vi "Initialize Time Tab.vi"(8 "error in (no error)":errorcluster, 11 "Numeric Data Type in":refnum<class "Numeric Data Type.lvclass">) -> (0 "error out":errorcluster, 3 "Numeric Data Type (dub)":refnum<class "Numeric Data Type.lvclass">)   [LabVIEW 2018, in "Numeric Data Type.lvclass"]
uses:
  Numeric Data Type.lvclass
  Numeric Data Type.lvclass/Numeric Data Type.ctl
  Reference Time Format.vi
  Reference Include Seconds.vi
  Reference HMS Digits.vi
  Reference Clock Type.vi
  Reference Date Format.vi
  Reference Date Order.vi
  Reference Year Format.vi
  Reference Display Type.vi
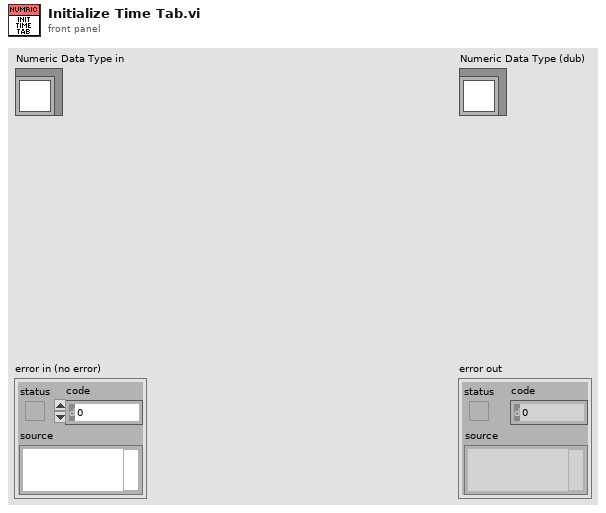
[diagram p1: front panel]
types:
  T1 = typedef "Numeric Data Type.lvclass/Time Info.ctl" = cluster{"Time Format":T2, "Numeric Format":T3, "Clock Type":T4, "Include Seconds?":bool, "Seconds Precision":i16, "Date Order":T5, "Date Format":T6, "Year Format":T7, "UTC":i16}
  T2 = typedef "Numeric Data Type.lvclass/Time Format.ctl" = enum16{"Custom time format", "System time format", "Time unused"}
  T3 = typedef "Numeric Data Type.lvclass/Numeric Format Enum.ctl" = enum16{"Floating Point Notation", "Scientific Notation", "Engineering Notation", "SI Notation", "<not used>", "Decimal", "Hexadecimal", "Octal", "Binary", "<not used 2>", "Absolute Time", "Relative Time"}
  T4 = typedef "Numeric Data Type.lvclass/Clock Type.ctl" = enum32{"12-Hour (AM/PM)", "24-Hour"}
  T5 = typedef "Numeric Data Type.lvclass/Date Order.ctl" = enum32{"M/D/Y", "D/M/Y", "Y/M/D"}
  T6 = typedef "Numeric Data Type.lvclass/Date Format.ctl" = enum16{"Custom date format", "System date format", "Date unused"}
  T7 = typedef "Numeric Data Type.lvclass/Year Format.ctl" = enum32{"No Year", "2-digit Year", "4-digit Year"}
  T8 = enum8{"Enabled", "Disabled", "Disabled and Grayed Out"}
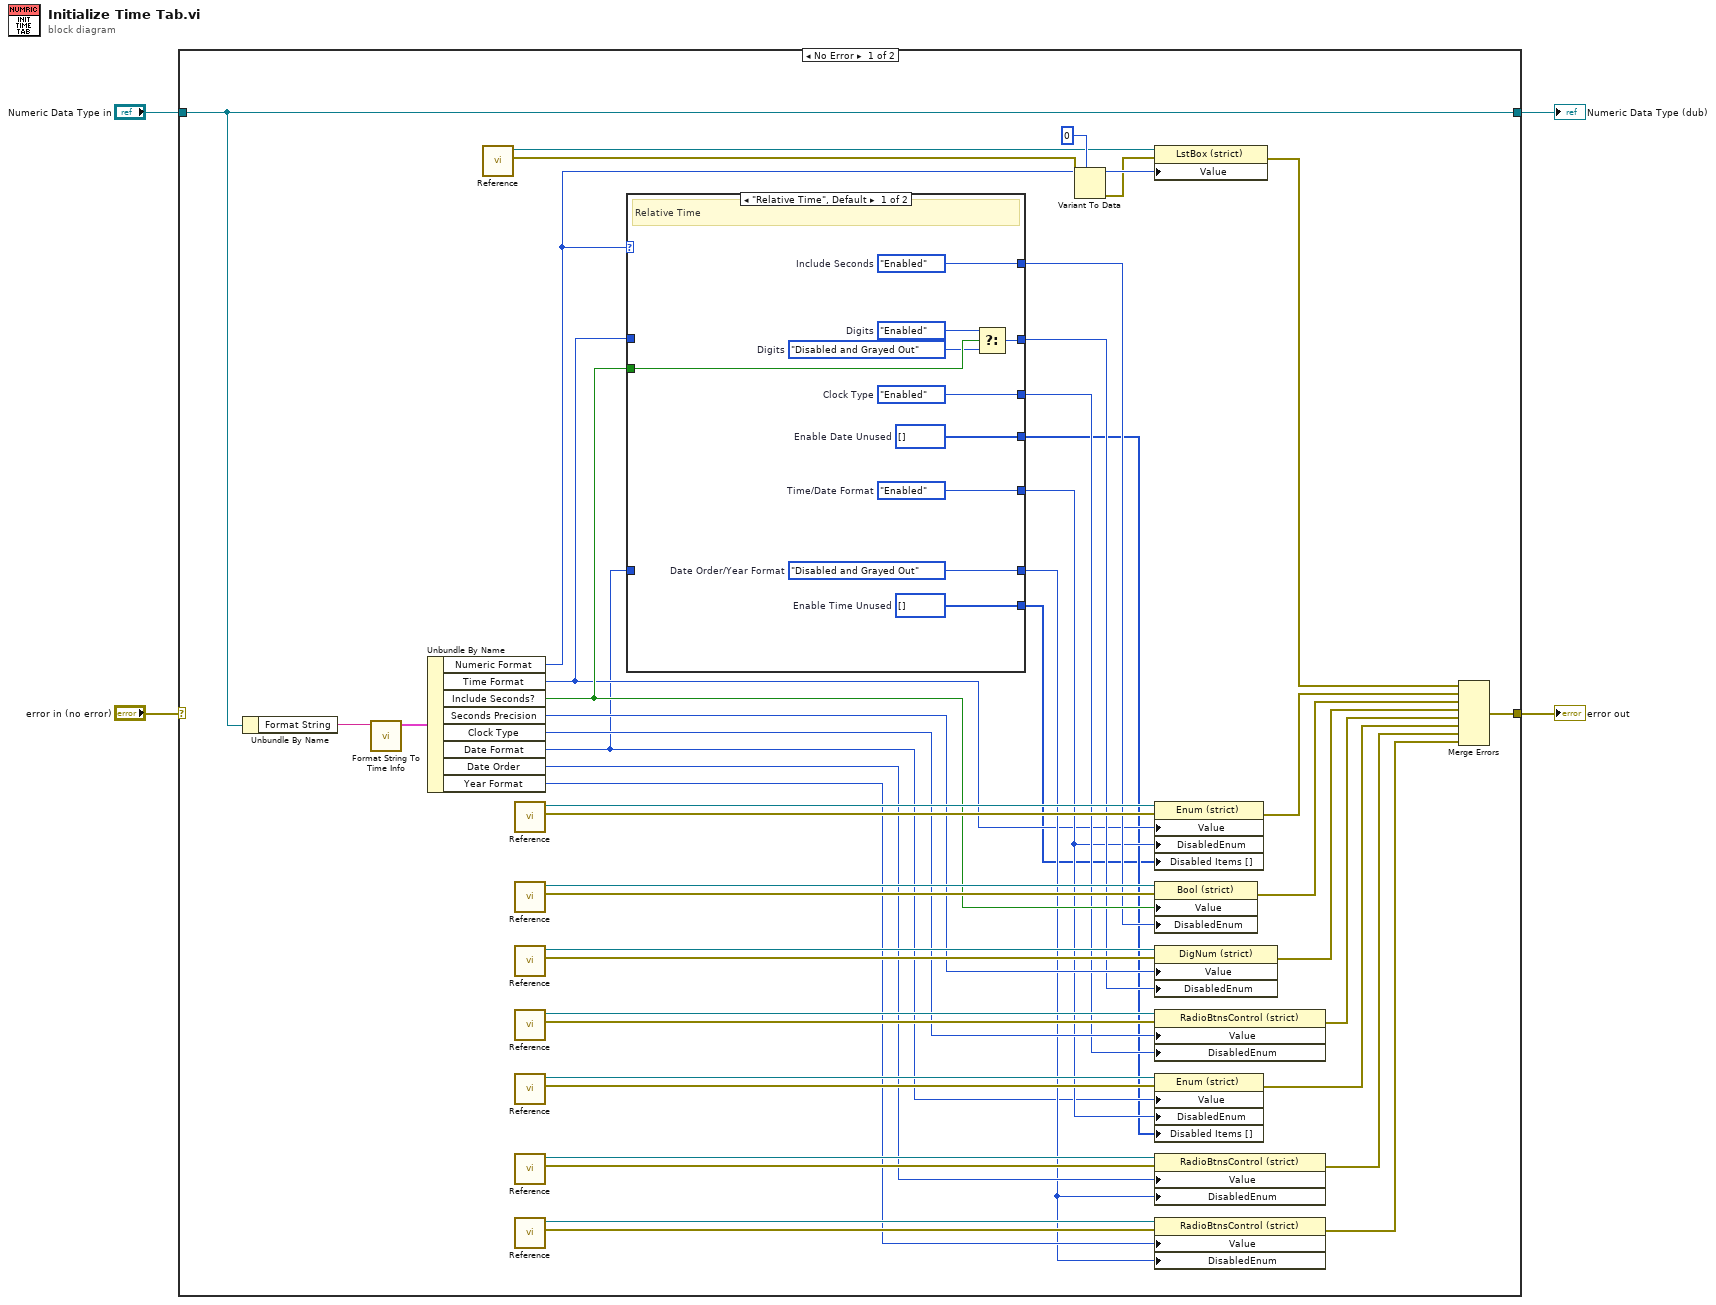
[diagram p0: block diagram]
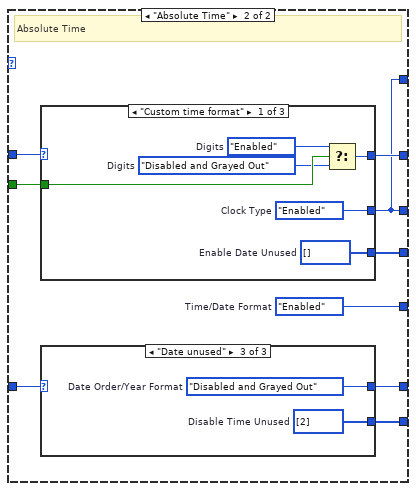
[diagram p2: hidden frame]
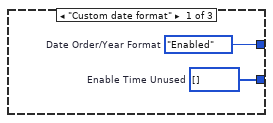
[diagram p3: hidden frame]
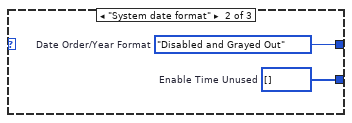
[diagram p4: hidden frame]
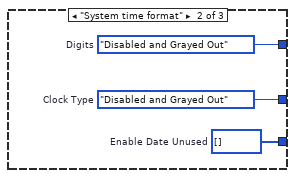
[diagram p5: hidden frame]
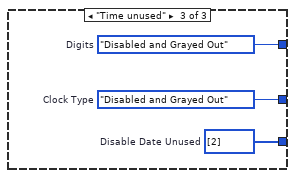
[diagram p6: hidden frame]
diagram:
  n1 = case shown="No Error" "error in (no error)" {
    selector: "error in (no error)" -> [_ w89]
    tunnel: [w28 w89] -> w3
    tunnel: [w50 w88] -> w1
    tunnel: "Numeric Data Type in" -> [w50 w88]
    frame No Error {
      n2 = Unbundle By Name(w50) -> ("Format String"=w49:string)
      n3 = call "Format String To Time Info.vi"("Format String"=w49) -> ("Time Info"=w48:T1)  [unwired: 10 in]
      n4 = Unbundle By Name(w48) -> ("Numeric Format"=w18:T3, "Time Format"=w8:T2, "Include Seconds?"=w16:bool, "Seconds Precision"=w41:i16, "Clock Type"=w38:T4, "Date Format"=w7:T6, "Date Order"=w11:T5, "Year Format"=w10:T7)
      n5 = call-poly "Reference.vi"() -> ("error out"=w20:errorcluster, "Display Type"=w29:refnum<vi>)  [unwired: 10 in]
      n6 = call-poly "Reference.vi"() -> ("error out"=w46:errorcluster, "Time Format"=w47:refnum<vi>)  [unwired: 10 in]
      n7 = call-poly "Reference.vi"() -> ("error out"=w44:errorcluster, "Include Seconds"=w45:refnum<vi>)  [unwired: 10 in]
      n8 = call-poly "Reference.vi"() -> ("error out"=w43:errorcluster, "HMS Digits"=w42:refnum<vi>)  [unwired: 10 in]
      n9 = call-poly "Reference.vi"() -> ("error out"=w39:errorcluster, "Clock Type"=w40:refnum<vi>)  [unwired: 10 in]
      n10 = call-poly "Reference.vi"() -> ("error out"=w37:errorcluster, "Date Format"=w36:refnum<vi>)  [unwired: 10 in]
      n11 = call-poly "Reference.vi"() -> ("error out"=w34:errorcluster, "Date Order"=w35:refnum<vi>)  [unwired: 10 in]
      n12 = call-poly "Reference.vi"() -> ("error out"=w33:errorcluster, "Year Format"=w32:refnum<vi>)  [unwired: 10 in]
      n13 = case shown="\"Relative Time\", Default" w18 {
        tunnel: [w59 w64] -> w13
        tunnel: [w60 w64] -> w14
        tunnel: w16 -> [w58 w69]
        tunnel: [w55 w68] -> w15
        tunnel: [w54 w67] -> w12
        tunnel: [w53 w66] -> w9
        tunnel: w8 -> [_ w65]
        tunnel: w7 -> [_ w63]
        tunnel: [w51 w62] -> w6
        tunnel: [w52 w61] -> w5
        frame "Relative Time", Default {
          w51 = i32[] []  # Enable Date Unused
          w52 = i32[] []  # Enable Time Unused
          w53 = T8."Disabled and Grayed Out"  # Date Order/Year Format
          w54 = T8."Enabled"  # Time/Date Format
          w56 = T8."Disabled and Grayed Out"  # Digits
          w57 = T8."Enabled"  # Digits
          w60 = T8."Enabled"  # Clock Type
          w59 = T8."Enabled"  # Include Seconds
          # "Relative Time"
          n14 = Select(t=w57, s=w58, f=w56) -> (s? t:f=w55:T8)
        }
        frame "Absolute Time" {
          w67 = T8."Enabled"  # Time/Date Format
          # "Absolute Time"
          n15 = case shown="\"Custom time format\"" w65 {
            tunnel: [w81 w84 w87] -> w64
            tunnel: w69 -> [w80 _ _]
            tunnel: [w77 w83 w86] -> w68
            tunnel: [w76 w82 w85] -> w62
            frame "Custom time format" {
              w76 = i32[] []  # Enable Date Unused
              w78 = T8."Disabled and Grayed Out"  # Digits
              w79 = T8."Enabled"  # Digits
              w81 = T8."Enabled"  # Clock Type
              n16 = Select(t=w79, s=w80, f=w78) -> (s? t:f=w77:T8)
            }
            frame "System time format" {
              w82 = i32[] []  # Enable Date Unused
              w83 = T8."Disabled and Grayed Out"  # Digits
              w84 = T8."Disabled and Grayed Out"  # Clock Type
            }
            frame "Time unused" {
              w85 = i32[] [2]  # Disable Date Unused
              w86 = T8."Disabled and Grayed Out"  # Digits
              w87 = T8."Disabled and Grayed Out"  # Clock Type
            }
          }
          n17 = case shown="\"Date unused\"" w63 {
            tunnel: [w71 w73 w75] -> w66
            tunnel: [w70 w72 w74] -> w61
            frame "Custom date format" {
              w70 = i32[] []  # Enable Time Unused
              w71 = T8."Enabled"  # Date Order/Year Format
            }
            frame "System date format" {
              w72 = i32[] []  # Enable Time Unused
              w73 = T8."Disabled and Grayed Out"  # Date Order/Year Format
            }
            frame "Date unused" {
              w74 = i32[] [2]  # Disable Time Unused
              w75 = T8."Disabled and Grayed Out"  # Date Order/Year Format
            }
          }
        }
      }
      n18 = Variant To Data(error in=w20, type=0, Variant=w18) -> (data=w30:i32, error out=w19:errorcluster)
      n19 = property class="LstBox (strict)"(reference=w29, error in=w19, "Value"=w30) -> (error out=w17:errorcluster)  [unwired: 1 out]
      n20 = property class="Enum (strict)"(reference=w47, error in=w46, "Value"=w8, "DisabledEnum"=w12, "Disabled Items []"=w5) -> (error out=w27:errorcluster)  [unwired: 1 out]
      n21 = property class="Bool (strict)"(reference=w45, error in=w44, "Value"=w16, "DisabledEnum"=w13) -> (error out=w26:errorcluster)  [unwired: 1 out]
      n22 = property class="DigNum (strict)"(reference=w42, error in=w43, "Value"=w41, "DisabledEnum"=w15) -> (error out=w25:errorcluster)  [unwired: 1 out]
      n23 = property class="RadioBtnsControl (strict)"(reference=w40, error in=w39, "Value"=w38, "DisabledEnum"=w14) -> (error out=w24:errorcluster)  [unwired: 1 out]
      n24 = property class="Enum (strict)"(reference=w36, error in=w37, "Value"=w7, "DisabledEnum"=w12, "Disabled Items []"=w6) -> (error out=w23:errorcluster)  [unwired: 1 out]
      n25 = property class="RadioBtnsControl (strict)"(reference=w35, error in=w34, "Value"=w11, "DisabledEnum"=w9) -> (error out=w22:errorcluster)  [unwired: 1 out]
      n26 = property class="RadioBtnsControl (strict)"(reference=w32, error in=w33, "Value"=w10, "DisabledEnum"=w9) -> (error out=w21:errorcluster)  [unwired: 1 out]
      n27 = Merge Errors(w17, w27, w26, w25, w24, w23, w22, w21) -> (w28:errorcluster)
    }
    frame Error {
    }
  }
  "error out" <- w3
  "Numeric Data Type (dub)" <- w1
